vi "readPinValYldrm.vi"(3 "YLDRMErrorInp":errorcluster, 4 "pin":u8, 5 "YLDRMPortInp":refnum<visa-resource-name>) -> (0 "YLDRMErrorOut":errorcluster, 1 "out":u8, 2 "YLDRMPortOut":refnum<visa-resource-name>)   [LabVIEW 2015]
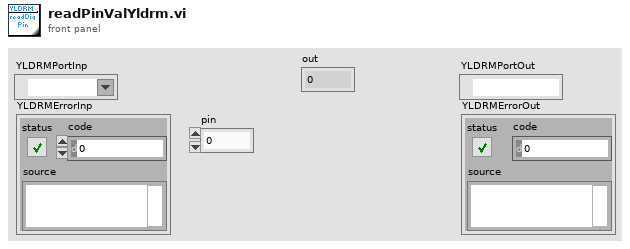
[diagram p1: front panel]
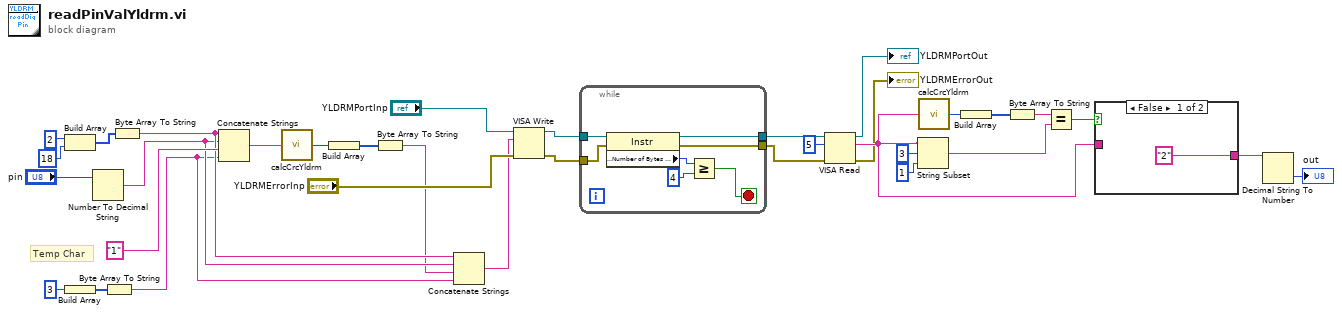
[diagram p0: block diagram]
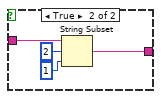
[diagram p2: hidden frame]
diagram:
  # "Temp Char"
  n1 = Build Array(2, 18) -> (w32:i32[])
  n2 = Build Array(3) -> (w29:i32[])
  n3 = Number To Decimal String(number="pin") -> (decimal integer string=w6:string)  [unwired: 1 in]
  n4 = Byte Array To String(unsigned byte array=w29) -> (string=w4:string)
  n5 = Byte Array To String(unsigned byte array=w32) -> (string=w7:string)
  n6 = Concatenate Strings(w7, w6, "1", w4) -> (w26:string)
  n7 = call "calcCrcYldrm.vi"("inpStr"=w26) -> ("crcVal"=w28:u8)
  n8 = Build Array(w28) -> (w27:u8[])
  n9 = Byte Array To String(unsigned byte array=w27) -> (string=w5:string)
  n10 = Concatenate Strings(w7, w6, w5, w4) -> (w3:string)
  n11 = VISA Write(VISA resource name="YLDRMPortInp", write buffer=w3, error in (no error)="YLDRMErrorInp") -> (VISA resource name out=w22:refnum<visa-resource-name>, error out=w21:errorcluster)  [unwired: 1 out]
  n12 = while {
    tunnel: w22 -> [w41]
    tunnel: w21 -> [w40]
    tunnel: [w39] -> w20
    tunnel: [w38] -> w19
    stop <- w35 stop-if-true
    n13 = property class="Instr"(reference=w41, error in=w40) -> (reference out=w39:refnum<visa-resource-name>, error out=w38:errorcluster, "Serial Settings:Number of Bytes at Serial Port"=w37:u32)
    n14 = Greater Or Equal?(x=w37, y=u32 4) -> (x >= y?=w35:bool)
  }
  n15 = VISA Read(VISA resource name=w20, byte count=u32 5, error in (no error)=w19) -> (VISA resource name out=→"YLDRMPortOut":refnum<visa-resource-name>, read buffer=w10:string, error out=→"YLDRMErrorOut":errorcluster)  [unwired: 1 out]
  n16 = String Subset(string=w10, offset (0)=3, length (rest)=1 ("length (rest)")) -> (substring=w12:string)
  n17 = call "calcCrcYldrm.vi"("inpStr"=w10) -> ("crcVal"=w16:u8)
  n18 = Build Array(w16) -> (w17:u8[])
  n19 = Byte Array To String(unsigned byte array=w17) -> (string=w13:string)
  n20 = Equal?(x=w13, y=w12) -> (x = y?=w11:bool)
  n21 = case shown="False" w11 {
    tunnel: w10 -> [_ w44]
    tunnel: ["2" w43] -> w2
    frame False {
    }
    frame True {
      n22 = String Subset(string=w44, offset (0)=2, length (rest)=1 ("length (rest)")) -> (substring=w43:string)
    }
  }
  n23 = Decimal String To Number(string=w2) -> (number=→"out":i32)  [unwired: 2 in, 1 out]
